vi "Init.vi"(8 "error in":errorcluster, 9 "Values":refnum<class "Value.lvclass">[](array[class]), 10 "Keys":refnum<class "Key Name.lvclass">[](array[class]), 11 "Object Type in":refnum<class "ARRAY.lvclass">) -> (0 "error out":errorcluster, 3 "Object Type out":refnum<class "ARRAY.lvclass">)   [LabVIEW 2020, in "Electronic Datasheet.lvlib" / "ARRAY.lvclass"]
uses:
  ARRAY.lvclass
  Keyname/Key Name.lvclass
  Value/Value.lvclass
  Object Type/Object Type Base.lvclass
  Electronic Datasheet.lvlib
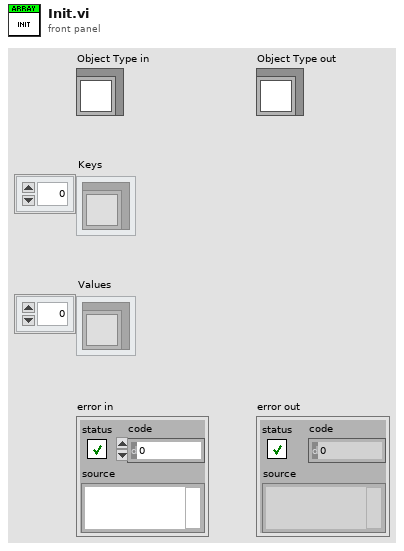
[diagram p1: front panel]
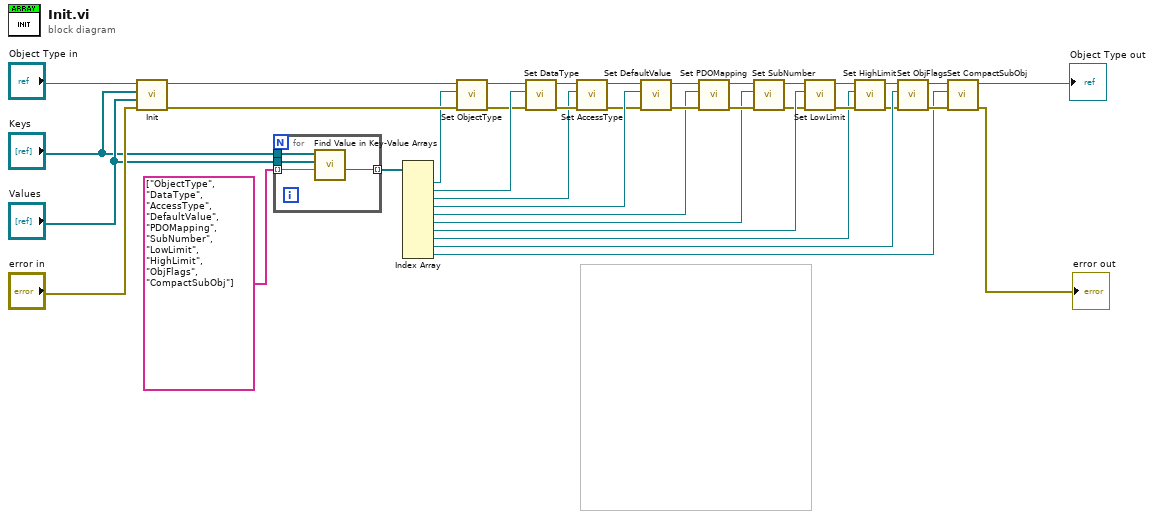
[diagram p0: block diagram]
diagram:
  n1 = call-parent "Init.vi"("error in"="error in", "Values"="Values", "Keys"="Keys", "Object Type in"="Object Type in") -> ("error out"=w37:errorcluster, "Object Type out"=w38:refnum<class "ARRAY.lvclass">)  [unwired: 6 in]
  n2 = for {
    tunnel: "Keys" -> [w42]
    tunnel: "Values" -> [w41]
    tunnel: [w40] -> w33 mode=indexing
    tunnel: string[] ["ObjectType", "DataType", "AccessType", "DefaultValue", "PDOMapping", "SubNumber", "LowLimit", "HighLimit", "ObjFlags", "CompactSubObj"] -> [w39] mode=indexing
    n3 = call "Find Value in Key-Value Arrays.vi"("Key Name"=w39, "Values"=w41, "Keys"=w42) -> ("Value"=w40:refnum<class "Value.lvclass">)  [unwired: 5 in, 3 out]
  }
  n4 = Index Array(array=w33) -> (element #1=w32:refnum<class "Value.lvclass">, element #2=w31:refnum<class "Value.lvclass">, element #3=w27:refnum<class "Value.lvclass">, element #4=w26:refnum<class "Value.lvclass">, element #5=w21:refnum<class "Value.lvclass">, element #6=w18:refnum<class "Value.lvclass">, element #7=w16:refnum<class "Value.lvclass">, element #8=w13:refnum<class "Value.lvclass">, element #9=w11:refnum<class "Value.lvclass">, element #10=w8:refnum<class "Value.lvclass">)  [unwired: 10 in]
  n5 = call-dynamic "Set ObjectType.vi"("error in"=w37, "ObjectType"=w32, "Object Type in"=w38) -> ("error out"=w29:errorcluster, "Object Type out"=w36:refnum<class "ARRAY.lvclass">)  [unwired: 7 in]
  n6 = call-dynamic "Set DataType.vi"("error in"=w29, "Value"=w31, "Object Type in"=w36) -> ("error out"=w28:errorcluster, "Object Type out"=w35:refnum<class "ARRAY.lvclass">)  [unwired: 7 in]
  n7 = call-dynamic "Set AccessType.vi"("error in"=w28, "Value"=w27, "Object Type in"=w35) -> ("error out"=w25:errorcluster, "Object Type out"=w30:refnum<class "ARRAY.lvclass">)  [unwired: 7 in]
  n8 = call-dynamic "Set DefaultValue.vi"("error in"=w25, "Value"=w26, "Object Type in"=w30) -> ("error out"=w22:errorcluster, "Object Type out"=w24:refnum<class "ARRAY.lvclass">)  [unwired: 7 in]
  n9 = call-dynamic "Set PDOMapping.vi"("error in"=w22, "Value"=w21, "Object Type in"=w24) -> ("error out"=w19:errorcluster, "Object Type out"=w23:refnum<class "ARRAY.lvclass">)  [unwired: 7 in]
  n10 = call-dynamic "Set SubNumber.vi"("error in"=w19, "Value"=w18, "Object Type in"=w23) -> ("error out"=w2:errorcluster, "Object Type out"=w20:refnum<class "ARRAY.lvclass">)  [unwired: 7 in]
  n11 = call-dynamic "Set LowLimit.vi"("error in"=w2, "Value.lvclass"=w16, "Object Type in"=w20) -> ("error out"=w14:errorcluster, "Object Type out"=w17:refnum<class "ARRAY.lvclass">)  [unwired: 7 in]
  n12 = call-dynamic "Set HighLimit.vi"("error in"=w14, "Value"=w13, "Object Type in"=w17) -> ("error out"=w1:errorcluster, "Object Type out"=w15:refnum<class "ARRAY.lvclass">)  [unwired: 7 in]
  n13 = call-dynamic "Set ObjFlags.vi"("error in"=w1, "Value"=w11, "Object Type in"=w15) -> ("error out"=w9:errorcluster, "Object Type out"=w12:refnum<class "ARRAY.lvclass">)  [unwired: 7 in]
  n14 = call-dynamic "Set CompactSubObj.vi"("error in"=w9, "Value"=w8, "Object Type in"=w12) -> ("error out"=→"error out":errorcluster, "Object Type out"=→"Object Type out":refnum<class "ARRAY.lvclass">)  [unwired: 7 in]
